vi "HEWH StateMachine.vi"() -> ()   [LabVIEW 2009]
panel:
  out "Error Out":errorcluster
  in  "Error In":errorcluster
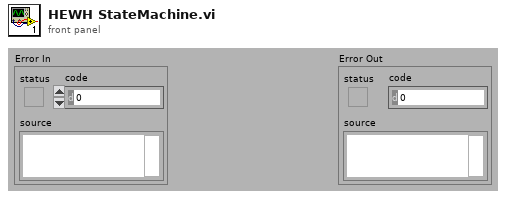
[diagram p1: front panel]
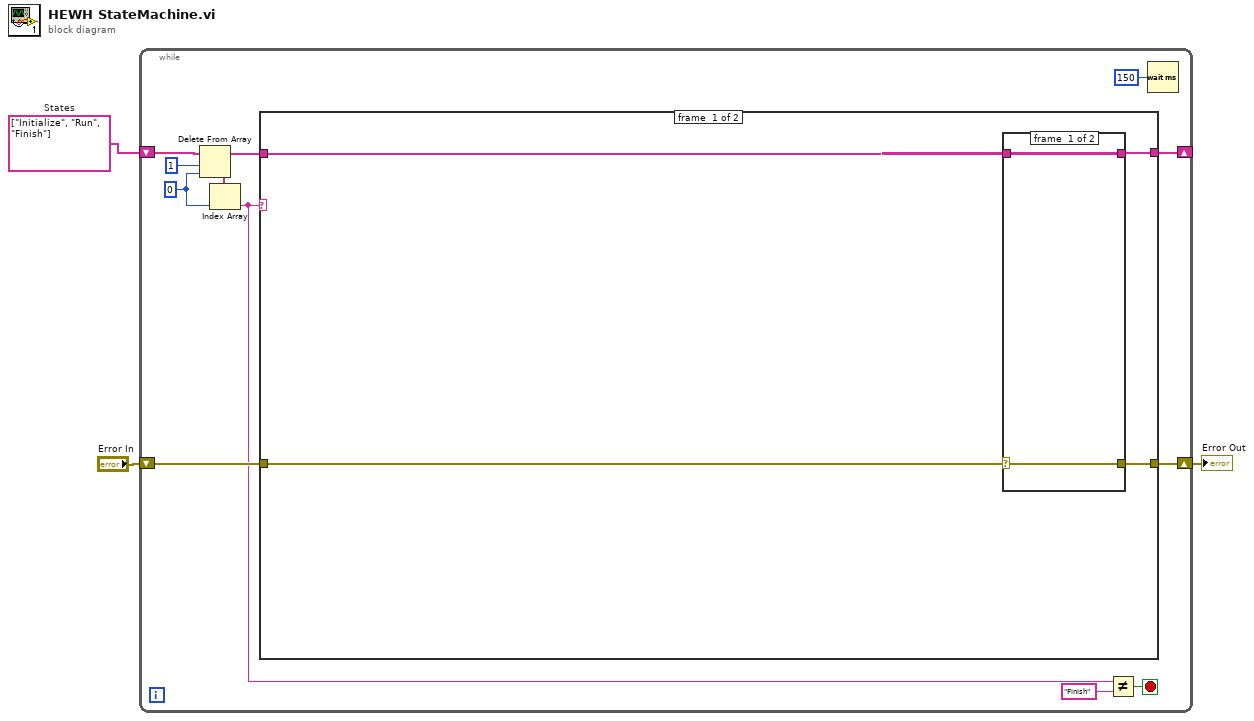
[diagram p0: block diagram]
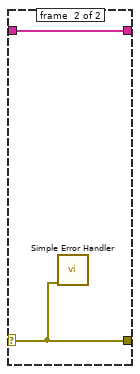
[diagram p2: hidden frame]
diagram:
  w3 = string[] ["Initialize", "Run", "Finish"]  # States
  n1 = while {
    shift-right: [w11] -> _
    shift-left: w3 -> [w15]
    shift-right: [w8] -> w1
    shift-left: "Error In" -> [w7]
    stop <- w6 stop-if-true
    w12 = 0 ("index")
    n2 = Delete From Array(array=w15, length=1, index=w12) -> (deleted portion=w13:string[], array with subset deleted=w10:string[])
    n3 = Index Array(array=w13, index=w12) -> (element=w5:string)
    n4 = case shown="\"Initialize\"" w5 {
      tunnel: [w19 w25] -> w11
      tunnel: w10 -> [w18 w25]
      tunnel: [w17 w24] -> w8
      tunnel: w7 -> [w16 w24]
      frame #0 {
        n5 = case shown="Error" w16 {
          selector: w16 -> [w20 w22]
          tunnel: [w21 w23] -> w19
          tunnel: w18 -> [w21 w23]
          tunnel: [w20 w22] -> w17
          frame #0 {
          }
          frame #1 {
            n6 = call <vilib>:"Simple Error Handler.vi"("error in (no error)"=w22) -> ()  [unwired: 4 in, 5 out]
          }
        }
      }
      frame #1 {
      }
    }
    n7 = Not Equal?(x=w5, y="Finish") -> (x != y?=w6:bool)
    n8 = Wait (ms)(milliseconds to wait=u32 150) -> ()  [unwired: 1 out]
  }
  "Error Out" <- w1
